vi "SaveLogData.vi"(8 "error in":errorcluster, 11 "File IO Data":T1={"System Log File"=path "", "Data File"=path "", "Work Order Folder"=path "", "Report Template Folder"=path "", "Report Folder"=path "", "Report File"=path "", "APU Setup Folder"=path "", "Testing State"=FALSE, "Recording State"=FALSE, "Test Information"={"APU Part Number:"="", "Model:"="", "Serial Number:"="", "Customer:"="", "Work Order:"="", "Pre or Post SB"="", "Run Count"=0, "APU Selected"="<Select>"}, "Crash Log Data"=[], "Group Name"="", "APU Setup"={"Sensor Info"=[], "Variables"=[], "CMM Table 106"=[], "CMM Table 106B "=[], "Accel Config"=[], "Report Sheet 1"=[], "Report Sheet 2"=[], "Report Sheet 3"=[]}, "ChannelTagsToLog"=[], "report ref"=refnum, "APU Setup File"=path "", "RunTimes"=[], "ReportHeader"=[]} {"Test Information"."Run Count" min=0 step=1}) -> (0 "error out":errorcluster)   [LabVIEW 2018, in "File IO.lvlib"]
uses:
  File IO.lvlib
  Private Controls/File IO Data.ctl
  <vilib>/Utility/NIReport.llb/NI_report.lvclass
  Controller (Host)/Public Controls/Test Information.ctl
  Controller (Host)/Public VIs/PreorPostSB.ctl
  Controller (Host)/Public Controls/APU Select.ctl
  Top Level/Shared Controls/Analyzed Data Sets.ctl
  Top Level/Shared Controls/All Data Cluster.ctl
  Top Level/Shared Controls/Acq Data.ctl
  Top Level/Shared Controls/APU Setup File.ctl
  <vilib>/Utility/file.llb/Write Delimited Spreadsheet (string).vi
  Controller (Host)/Controller (Host).lvlib
panel:
  out "Values":dbl[](array[numeric])
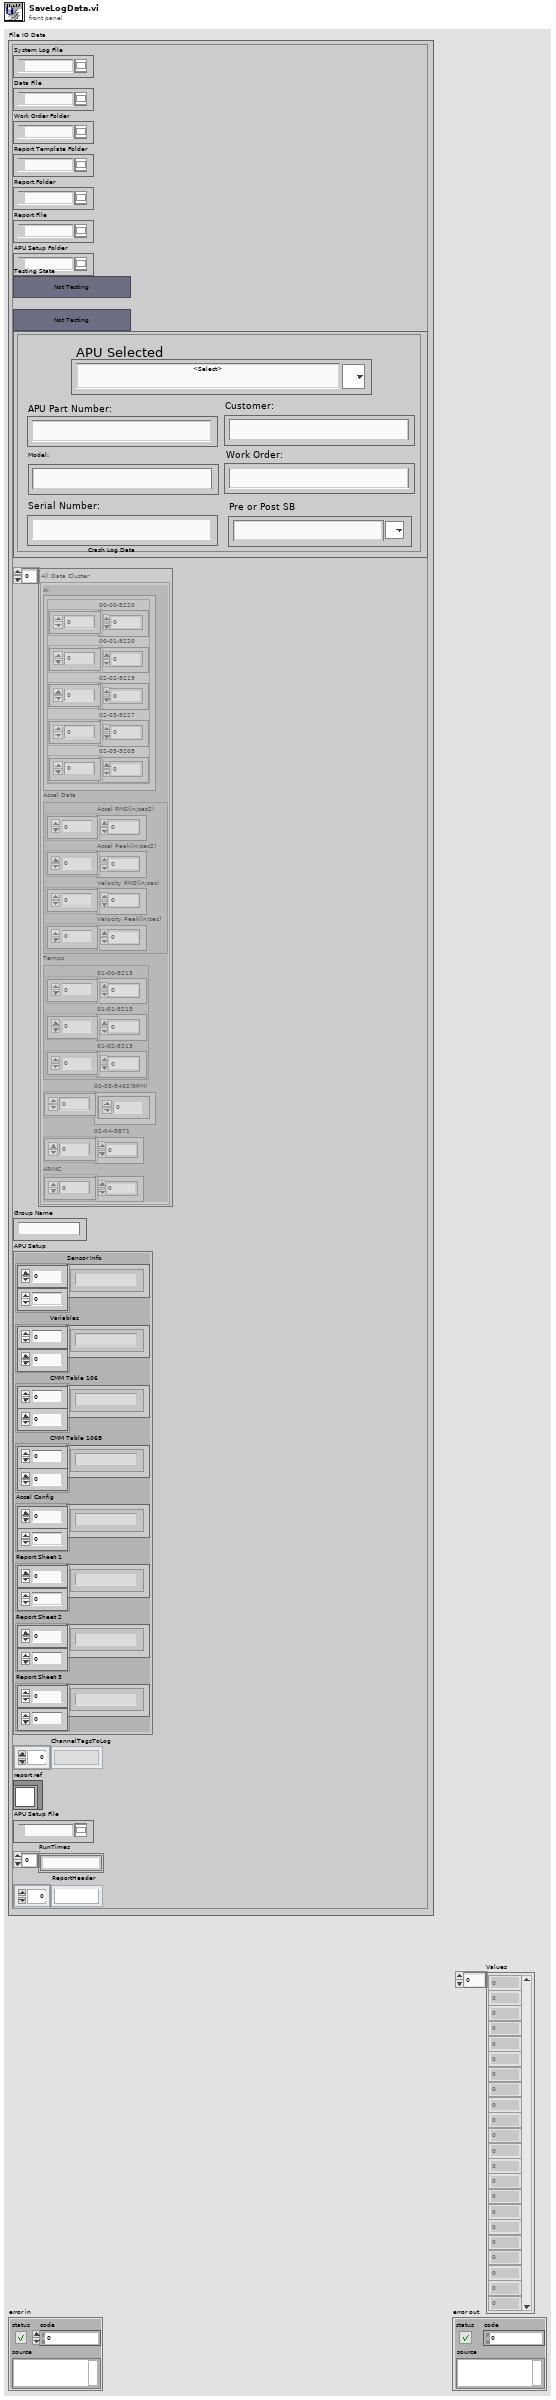
[diagram p1: front panel]
types:
  T1 = typedef "File IO.lvlib/File IO Data.ctl" = cluster{"System Log File":path, "Data File":path, "Work Order Folder":path, "Report Template Folder":path, "Report Folder":path, "Report File":path, "APU Setup Folder":path, "Testing State":bool, "Recording State":bool, "Test Information":T2, "Crash Log Data":T5, "Group Name":string, "APU Setup":T8, "ChannelTagsToLog":string[], "report ref":refnum<class "NI_report.lvclass">, "APU Setup File":path, "RunTimes":string[], "ReportHeader":string[]}
  T2 = typedef "Controller (Host).lvlib/Test Information.ctl" = cluster{"APU Part Number:":string, "Model:":string, "Serial Number:":string, "Customer:":string, "Work Order:":string, "Pre or Post SB":T3, "Run Count":i32, "APU Selected":T4}
  T3 = typedef "Controller (Host).lvlib/PreorPostSB.ctl" = string
  T4 = typedef "Controller (Host).lvlib/APU Select.ctl" = string
  T5 = typedef "Analyzed Data Sets.ctl" = T6[]
  T6 = typedef "All Data Cluster.ctl" = cluster{"AI":T7, "Accel Data":cluster{"Accel RMS(in/sec2)":dbl[], "Accel Peak(in/sec2)":dbl[], "Velocity RMS(in/sec)":dbl[], "Velocity Peak(in/sec)":dbl[]}, "Temps":cluster{"01-00-9213":dbl[], "01-01-9213":dbl[], "01-02-9213":dbl[]}, "00-03-9402(RPM)":dbl[], "02-04-9871":dbl[], "ARINC":sgl[]}
  T7 = typedef "Acq Data.ctl" = cluster{"00-00-9220":dbl[], "00-01-9220":dbl[], "02-02-9219":dbl[], "02-03-9227":dbl[], "02-05-9205":dbl[]}
  T8 = typedef "APU Setup File.ctl" = cluster{"Sensor Info":string[][], "Variables":string[][], "CMM Table 106":string[][], "CMM Table 106B ":string[][], "Accel Config":string[][], "Report Sheet 1":string[][], "Report Sheet 2":string[][], "Report Sheet 3":string[][]}
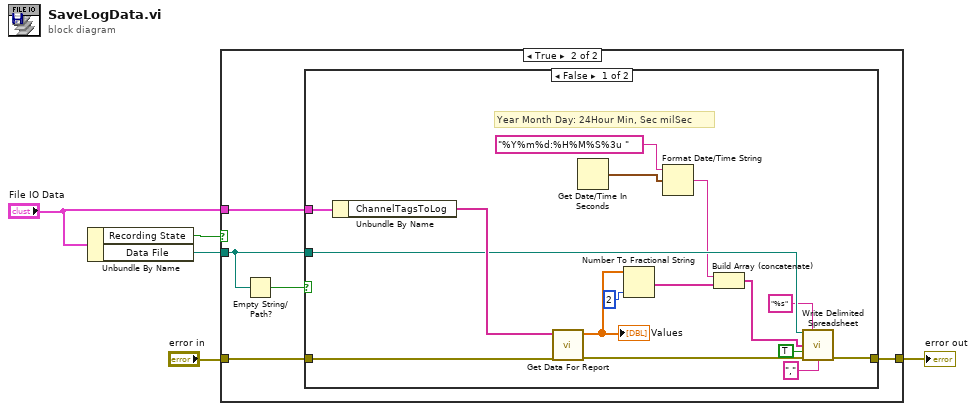
[diagram p0: block diagram]
diagram:
  n1 = Unbundle By Name("File IO Data") -> ("Recording State"=w1:bool, "Data File"=w4:path)
  n2 = case shown="True" w1 {
    tunnel: "error in" -> [w6 w9]
    tunnel: [w6 w8] -> w3
    tunnel: w4 -> [_ w7]
    tunnel: "File IO Data" -> [_ w10]
    frame False {
    }
    frame True {
      n3 = Empty String/Path?(string/path=w7) -> (empty?=w11:bool)
      n4 = case shown="False" w11 {
        tunnel: w10 -> [w27 _]
        tunnel: w9 -> [w25 w28]
        tunnel: [w22 w28] -> w8
        tunnel: w7 -> [w24 _]
        frame False {
          # "Year Month Day: 24Hour Min, Sec milSec"
          n5 = Unbundle By Name(w27) -> ("ChannelTagsToLog"=w26:string[])
          n6 = call "Get Data For Report.vi"("error constant"=w25, "Channel Tags"=w26) -> ("error out"=w23:errorcluster, "Value"=w19:dbl[])  [unwired: 8 in]
          "Values" <- w19
          n7 = Get Date/Time In Seconds() -> (seconds since 1Jan1904=w14:timestamp)
          n8 = Number To Fractional String(number=w19, precision (6)=i16 2) -> (F-format string=w17:string[])  [unwired: 2 in]
          n9 = Format Date/Time String(time format string (%c)="%Y%m%d:%H%M%S%3u ", seconds (now)=w14) -> (date/time string=w13:string)  [unwired: 1 in]
          n10 = Build Array (concatenate)(w13, w17) -> (w15:string[])
          n11 = call-poly <vilib>:"Write Delimited Spreadsheet.vi"("file path (dialog if empty)"=w24, "format (%s)"="%s" ("format (%.3f)"), "1D data"=w15, "append to file? (new file:F)"=TRUE, "error in (no error)"=w23, "delimiter (\\t)"="," ("delimiter (\\t)")) -> ("error out"=w22:errorcluster)  [unwired: 8 in, 1 out]
        }
        frame True {
          # "No Active Test. Ignore"
        }
      }
    }
  }
  "error out" <- w3
